vi "Autosampler Move Needle.vi"(7 "Correlation ID":u32, 8 "error in (no error)":errorcluster, 10 "Needle Position":T1, 11 "Application in":refnum<class "Application.lvclass">) -> (0 "error out":errorcluster, 3 "Application out":refnum<class "Application.lvclass">)   [LabVIEW 2023, in "Application.lvlib" / "Application.lvclass"]
uses:
  Application.lvclass
  Hardware/Autosampler/Autosampler Needle Position.ctl
  Application.lvclass/Application.ctl
  Hardware/Device Messages/Save CorrID Msg/Save CorrID Msg.lvclass/Save CorrID Msg.ctl
  <vilib>/ActorFramework/Message Enqueuer/Message Enqueuer.lvclass/Message Enqueuer.ctl
  Hardware/Autosampler Messages/Move Needle Msg/Move Needle Msg.lvclass/Move Needle Msg.ctl
  <vilib>/ActorFramework/Message Enqueuer/Enqueue.vi
  Hardware/Device Messages/Save CorrID Msg/Save CorrID Msg.lvclass
  C:/Program Files/National Instruments/LabVIEW 2023/vi.lib/ActorFramework/Message/Message.lvclass
  Hardware/Autosampler Messages/Move Needle Msg/Move Needle Msg.lvclass
  <vilib>/ActorFramework/Message Priority Queue/Priority Enqueue.vi
  Hardware/Autosampler/Autosampler.lvlib
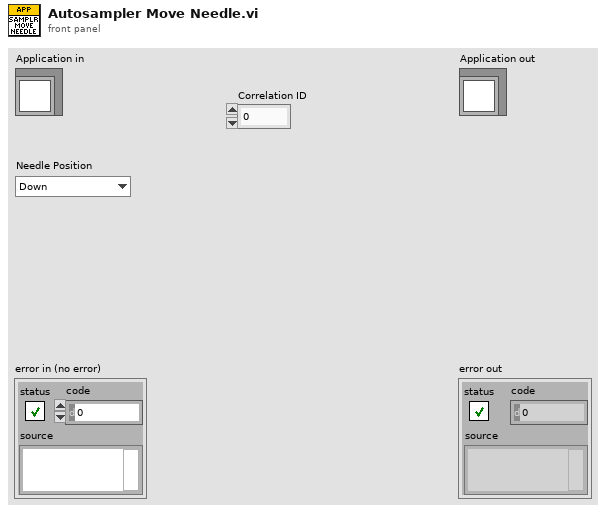
[diagram p1: front panel]
types:
  T1 = typedef "Autosampler.lvlib/Autosampler Needle Position.ctl" = enum16{"Down", "Up"}
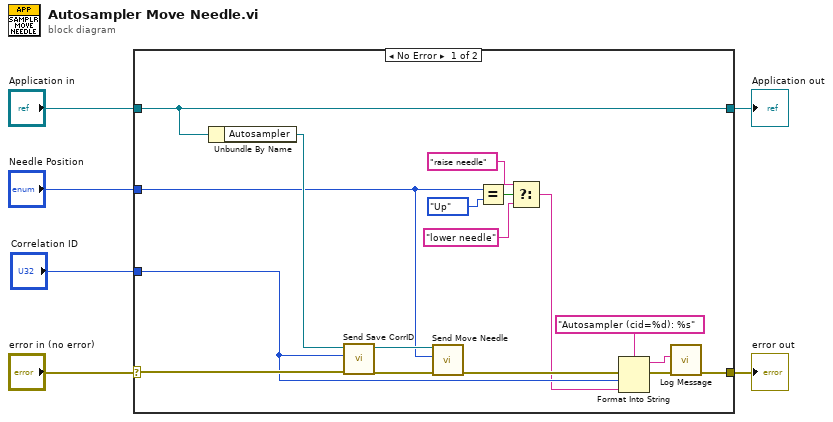
[diagram p0: block diagram]
diagram:
  n1 = case shown="No Error" "error in (no error)" {
    selector: "error in (no error)" -> [w21 w25]
    tunnel: [w18 w25] -> w5
    tunnel: [w23 w24] -> w3
    tunnel: "Application in" -> [w23 w24]
    tunnel: "Needle Position" -> [w15 _]
    tunnel: "Correlation ID" -> [w11 _]
    frame No Error {
      n2 = Unbundle By Name(w23) -> ("Autosampler"=w20:refnum<class "Message Enqueuer.lvclass">)
      n3 = call "Send Save CorrID.vi"("error in (no error)"=w21, "Correlation ID"=w11, "Message Enqueuer"=w20) -> ("error out"=w22:errorcluster, "Message Enqueuer out"=w19:refnum<class "Message Enqueuer.lvclass">)  [unwired: 7 in]
      n4 = call "Send Move Needle.vi"("error in (no error)"=w22, "Needle Position"=w15, "Message Enqueuer"=w19) -> ("error out"=w10:errorcluster)  [unwired: 7 in, 1 out]
      n5 = Equal?(x=w15, y=Autosampler_Needle_Position."Up") -> (x = y?=w16:bool)
      n6 = Select(t="raise needle", s=w16, f="lower needle") -> (s? t:f=w8:string)
      n7 = Format Into String(format string="Autosampler (cid=%d): %s" ("string"), error in=w10, w11, w8) -> (resulting string=w7:string, error out=w9:errorcluster)  [unwired: 1 in]
      n8 = call "Log Message.vi"("error constant"=w9, "input"=w7) -> ("error constant 2"=w18:errorcluster)  [unwired: 8 in, 1 out]
    }
    frame Error {
    }
  }
  "error out" <- w5
  "Application out" <- w3
